vi "Sub Initialize.vi"(6 "Controller name":string, 8 "error in (no error)":errorcluster, 11 "Instrument Recorder in":refnum<class "Lockin Digitizer.lvclass">) -> (0 "error out":errorcluster, 2 "Initialize Result":refnum<class "Acquired Result.lvclass">, 3 "Instrument Recorder out":refnum<class "Lockin Digitizer.lvclass">)   [LabVIEW 2021, in "Lockin Digitizer.lvclass"]
uses:
  Lockin Digitizer.lvclass
  NHMFL_Core/Libraries/Instruments/Results/Acquired Result/Acquired Result.lvclass
  NHMFL_Core/Libraries/Instruments/Results/Acquired Result/Acquired Result.lvclass/Acquired Result.ctl
  NHMFL_Core/Libraries/Instruments/Results/Acquired Result/Write Channels.vi
  NHMFL_Core/Libraries/Instruments/Pulse Driver/Lockin Digitizer Driver/Lockin Digitizer Driver.lvclass
  Pulse Recorder Actor/Pulse Recorder Actor.lvclass
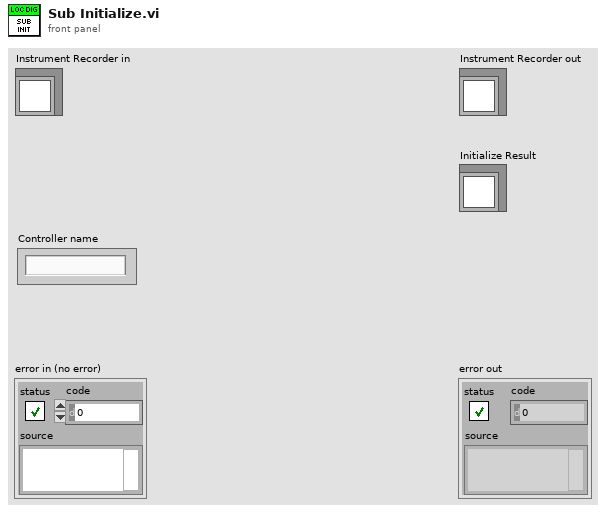
[diagram p1: front panel]
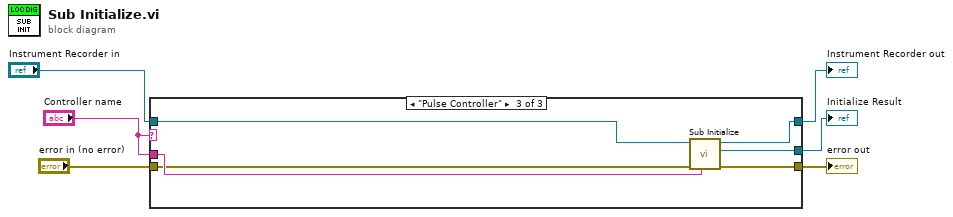
[diagram p0: block diagram]
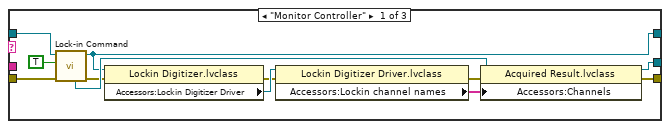
[diagram p2: hidden frame]
diagram:
  n1 = case shown="\"Pulse Controller\"" "Controller name" {
    tunnel: "Controller name" -> [_ _ w26]
    tunnel: "error in (no error)" -> [w15 w20 w25]
    tunnel: "Instrument Recorder in" -> [w16 w19 w24]
    tunnel: [w14 w20 w23] -> w3
    tunnel: [w13 _ w22] -> w2
    tunnel: [w12 w19 w21] -> w1
    frame "Monitor Controller" {
      n2 = call-dynamic "Lock-in Command.vi"("error in (no error)"=w15, "Lock-in"=TRUE, "Lockin Digitizer in"=w16) -> ("error out"=w8:errorcluster, "Lockin Digitizer out"=w12:refnum<class "Lockin Digitizer.lvclass">, "Result"=w17:refnum<class "Acquired Result.lvclass">)  [unwired: 6 in]
      n3 = property class="Lockin Digitizer.lvclass"(reference=w12, error in=w8) -> (error out=w9:errorcluster, "Accessors:Lockin Digitizer Driver"=w11:refnum<class "Lockin Digitizer Driver.lvclass">)  [unwired: 1 out]
      n4 = property class="Lockin Digitizer Driver.lvclass"(reference=w11, error in=w9) -> (error out=w7:errorcluster, "Accessors:Lockin channel names"=w10:string[])  [unwired: 1 out]
      n5 = property class="Acquired Result.lvclass"(reference=w17, error in=w7, "Accessors:Channels"=w10) -> (reference out=w13:refnum<class "Acquired Result.lvclass">, error out=w14:errorcluster)
    }
    frame "none", Default {
    }
    frame "Pulse Controller" {
      n6 = call-parent "Sub Initialize.vi"("Controller name"=w26, "error in (no error)"=w25, "Instrument Recorder in"=w24) -> ("error out"=w23:errorcluster, "Initialize Result"=w22:refnum<class "Acquired Result.lvclass">, "Instrument Recorder out"=w21:refnum<class "Lockin Digitizer.lvclass">)  [unwired: 6 in]
    }
  }
  "error out" <- w3
  "Instrument Recorder out" <- w1
  "Initialize Result" <- w2
